vi "izaberi_sliku_kapsule.vi"(8 "error in":errorcluster, 10 "Izbor kafe ulaz":T1) -> (0 "error out":errorcluster, 1 "prekinut":bool, 2 "Izbor kafe izlaz":T1)   [LabVIEW 2019]
doc: "Od korisnika se zahteva izbor slike. Proverava se da li je slika u skladu sa izborom kafe sa ulaza. Slika se upoređuje po boji sa poznatim slikama kapsula. Ako je izabrana slika odgovarajuća prosleđuje se isti izbor na izlaz. Ako slika nije odgovarajuća šalje se greška."
uses:
  vrste_kafe.ctl
panel:
  out "max index(es)":i32[](array[numeric])
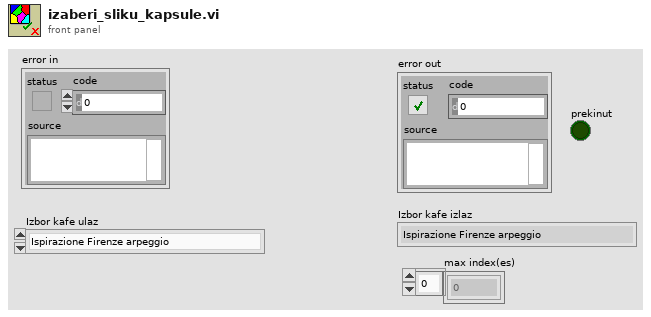
[diagram p1: front panel]
types:
  T1 = typedef "vrste_kafe.ctl" = enum16{"Ispirazione Firenze arpeggio", "Barista Corto", "Ispirazione Napoli"}
  T2 = typedef "IMAQ Image.ctl" = refnum<image>
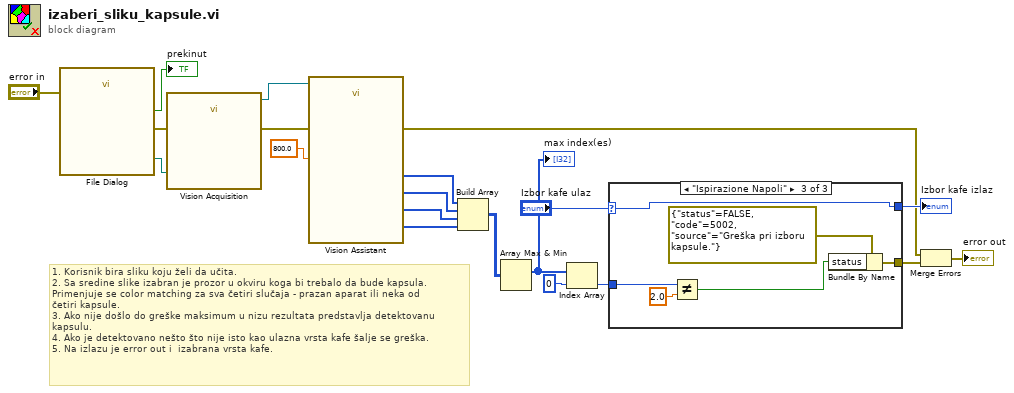
[diagram p0: block diagram]
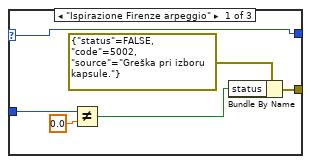
[diagram p2: hidden frame]
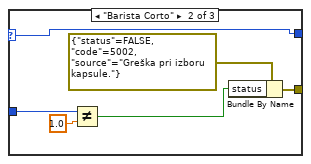
[diagram p3: hidden frame]
diagram:
  # "1. Korisnik bira sliku koju želi da učita.\n2. Sa sredine slike izabran je prozor u okviru koga bi trebalo da bude kapsula.\nPrimenjuje se color matching za sva četiri slučaja - prazan aparat ili neka od\nčetiri kapsule. \n3. Ako nije došlo do greške maksimum u nizu rezultata predstavlja detektovanu\nkapsulu.\n4. Ako je detektovano nešto što nije isto kao ulazna vrsta kafe šalje se greška.\n5. Na izlazu je error out i  izabrana vrsta kafe."
  n1 = call "File Dialog"("error in"="error in") -> ("selected path"=w20:path, "cancelled"=→"prekinut":bool, "error out"=w19:errorcluster)  [unwired: 11 in, 1 out]
  n2 = call "Vision Acquisition"("Image Path"=w20, "error in"=w19) -> ("Image Out"=w17:T2, "error out"=w16:errorcluster)  [unwired: 24 in]
  n3 = call "Vision Assistant"("Image In"=w17, "Minimum Match Score (Color Matching 1)"=800.0, "error in"=w16) -> ("Match Score (Color Matching 2)"=w8:i32[], "Match Score (Color Matching 1)"=w9:i32[], "Match Score (Color Matching 3)"=w7:i32[], "Match Score (Color Matching 4)"=w6:i32[], "error out"=w4:errorcluster)  [unwired: 19 in, 1 out]
  n4 = Build Array(w9, w8, w7, w6) -> (w2:i32[][])
  n5 = Array Max & Min(array=w2) -> (max index (indices)=w1:i32[])  [unwired: 3 out]
  "max index(es)" <- w1
  n6 = Index Array(array=w1, index=0) -> (element=w12:i32)
  n7 = case shown="\"Ispirazione Napoli\"" "Izbor kafe ulaz" {
    selector: "Izbor kafe ulaz" -> [w25 w29 w35]
    tunnel: w12 -> [w21 w27 w33]
    tunnel: [w25 w29 w35] -> w13
    tunnel: [w23 w28 w34] -> w3
    frame "Ispirazione Firenze arpeggio" {
      n8 = Not Equal?(x=w21, y=0.0) -> (x != y?=w22:bool)
      n9 = Bundle By Name(cluster=errorcluster {"status"=FALSE, "code"=5002, "source"="Greška pri izboru kapsule."} ("error constant"), "status"=w22) -> (w23:errorcluster)
    }
    frame "Barista Corto" {
      n10 = Not Equal?(x=w27, y=1.0) -> (x != y?=w30:bool)
      n11 = Bundle By Name(cluster=errorcluster {"status"=FALSE, "code"=5002, "source"="Greška pri izboru kapsule."} ("error constant"), "status"=w30) -> (w28:errorcluster)
    }
    frame "Ispirazione Napoli" {
      n12 = Not Equal?(x=w33, y=2.0) -> (x != y?=w36:bool)
      n13 = Bundle By Name(cluster=errorcluster {"status"=FALSE, "code"=5002, "source"="Greška pri izboru kapsule."} ("error constant"), "status"=w36) -> (w34:errorcluster)
    }
  }
  "Izbor kafe izlaz" <- w13
  n14 = Merge Errors(w4, w3) -> (→"error out":errorcluster)
